vi "Terminal_Voice_Signal_Processing.vi"(0 "输入信号":dbl[](array[numeric])=[0.0, 1.0, 3.0, 1.0, 2.0, 0.0, 4.0, 3.0, 5.0, 2.0, 1.0, 0.0, 4.0, 5.0, 1.0, 2.0, 3.0] caption="X", 5 "阈值":dbl format="%0.2f") -> (3 "事件计数":i32, 4 "振铃计数":i32, 8 "幅值":dbl, 10 "RMS":dbl, 14 "能量":dbl, 15 "RMS value":dbl caption="均方根值" format="%0.5f")   [LabVIEW 2014]
uses:
  <vilib>/measure/madcrms.llb/Basic Averaged DC-RMS for 1 Chan.vi
  <vilib>/Analysis/NI_AAL_SigProc.lvlib
  <vilib>/measure/NI_MAPro.lvlib
panel:
  out "数组":dbl[](array[numeric])
  out "信号波形图":dbl[](graph)
  # "声发射信号分析"
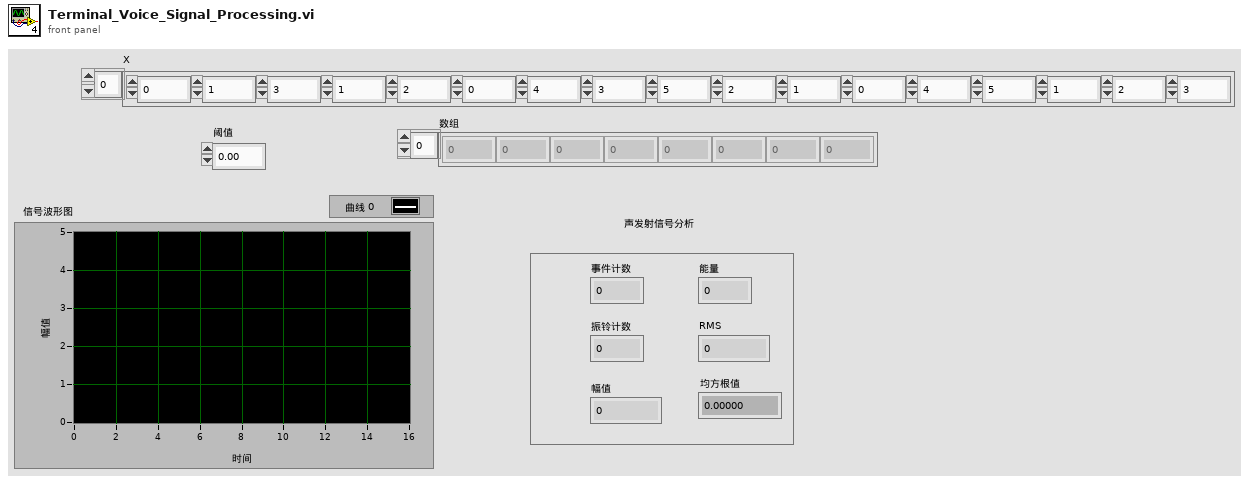
[diagram p1: front panel]
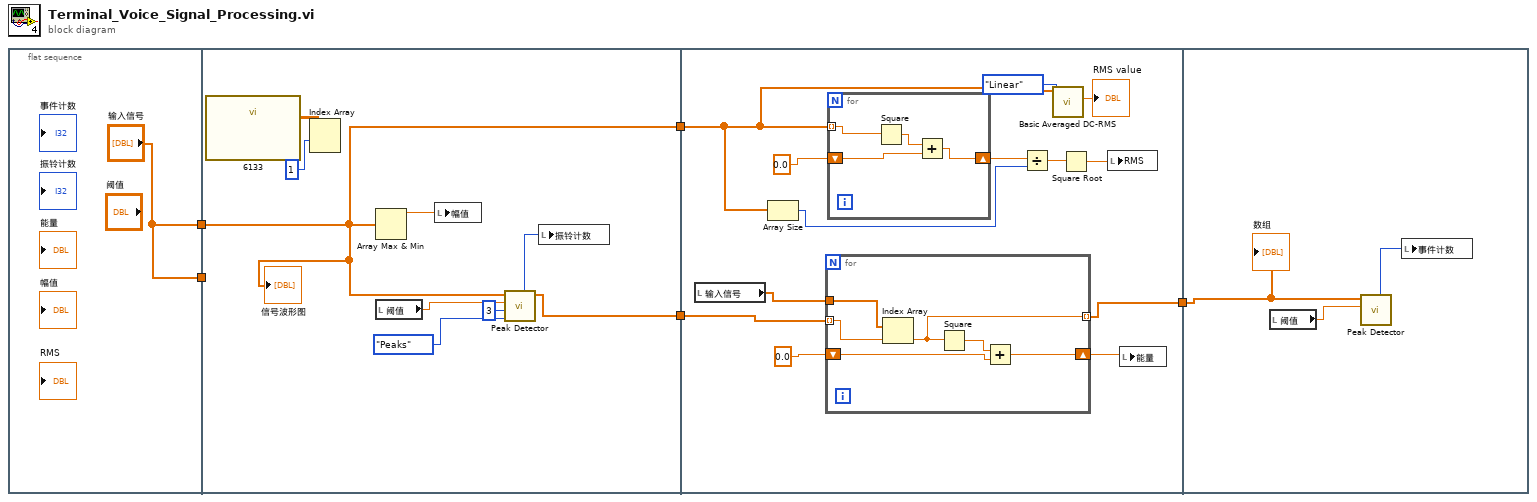
[diagram p0: block diagram]
diagram:
  n1 = flat-sequence {
    tunnel: ["输入信号"] -> w2
    tunnel: ["输入信号"] -> w1
    tunnel: [w11] -> w5
    tunnel: [w7] -> w3
    tunnel: w2 -> [w7]
    tunnel: w1 -> [_]
    tunnel: w5 -> [w27]
    tunnel: [w24] -> w4
    tunnel: w3 -> [w18]
    tunnel: w4 -> [w40]
    frame #0 {
    }
    frame #1 {
      n2 = call "6133.vi"() -> ("data"=w10:sgl[][])  [unwired: 16 in, 3 out]
      n3 = Index Array(array=w10, index (row)=1 ("禁用的索引 (列)")) -> ()  [unwired: 1 in, 1 out]
      n4 = Array Max & Min(array=w7) -> (max value=w12:dbl)  [unwired: 3 out]
      n5 = local read "阈值"() -> (w14:dbl)
      n6 = local write "幅值"(w12) -> ()
      n7 = call <vilib>:"Peak Detector.vi"("peaks/valleys"=enum32{"Peaks", "Valleys"}."Peaks", "width"=3, "threshold"=w14, "X"=w7) -> ("Locations"=w11:dbl[], "# found"=w13:i32)  [unwired: 3 in, 3 out]
      n8 = local write "振铃计数"(w13) -> ()
      "信号波形图" <- w7
    }
    frame #2 {
      n9 = local read "输入信号"() -> (w28:dbl[])
      n10 = Array Size(array=w18) -> (size(s)=w21:i32)
      n11 = for {
        tunnel: w28 -> [w33]
        tunnel: w27 -> [w38] mode=indexing
        shift-right: [w35] -> w25
        shift-left: 0.0 -> [w36]
        tunnel: [w34] -> w24 mode=indexing
        n12 = Index Array(array=w33, index=w38) -> (element=w34:dbl)
        n13 = Square(x=w34) -> (x^2=w37:dbl)
        n14 = Add(x=w37, y=w36) -> (x+y=w35:dbl)
      }
      n15 = for {
        tunnel: w18 -> [w32] mode=indexing
        shift-right: [w29] -> w22
        shift-left: 0.0 -> [w30]
        n16 = Square(x=w32) -> (x^2=w31:dbl)
        n17 = Add(x=w31, y=w30) -> (x+y=w29:dbl)
      }
      n18 = Divide(x=w22, y=w21) -> (x/y=w20:dbl)
      n19 = call-poly <vilib>:"Basic Averaged DC-RMS.vi"("averaging type"=enum16{"Linear", "Exponential"}."Linear", "signal in"=w18) -> ("RMS value"=→"RMS value":dbl)  [unwired: 6 in, 3 out]
      n20 = Square Root(x=w20) -> (sqrt(x)=w19:dbl)
      n21 = local write "RMS"(w19) -> ()
      n22 = local write "能量"(w25) -> ()
    }
    frame #3 {
      n23 = local read "阈值"() -> (w39:dbl)
      n24 = call <vilib>:"Peak Detector.vi"("threshold"=w39, "X"=w40) -> ("# found"=w41:i32)  [unwired: 5 in, 4 out]
      n25 = local write "事件计数"(w41) -> ()
      "数组" <- w40
    }
  }
